vi "CalcParams.vi"(0 "Max":sgl, 5 "ClkRate":sgl, 7 "fc":sgl, 9 "deadtime":sgl) -> (4 "Parameters":T1={"max"=0.9999695, "Period"=0, "Deadtime"=1})   [LabVIEW 2015, in "SVPWMInterface.lvlib"]
doc: "Calculates parameters nescessary to configure the SPWM Core.\n\nClkRate - The clock rate in Hz that the core will execute at, typically determined by the clock rate of a single cycle timed loop. Typical values would be 40 MHz or 80 MHz. Recommended values would be 10 to 20 kHz.\n\nfc - Carrier frequency in Hz of the PWM. Recommended values would be 10 kHz to 20 kHz.\n\nDeadtime - Deadtime between switching between the Top and Bottom switch pairs in seconds."
uses:
  SVPWMInterface.lvlib
  SVPWM/SVPWM_SGL.ctl
  SVPWM/SVPWM.lvlib
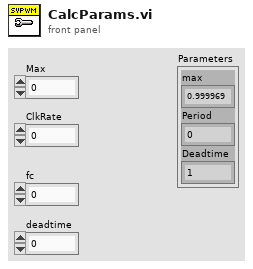
[diagram p1: front panel]
types:
  T1 = typedef "SVPWM.lvlib/SVPWM_SGL.ctl" = cluster{"max":sgl, "Period":u32, "Deadtime":u8}
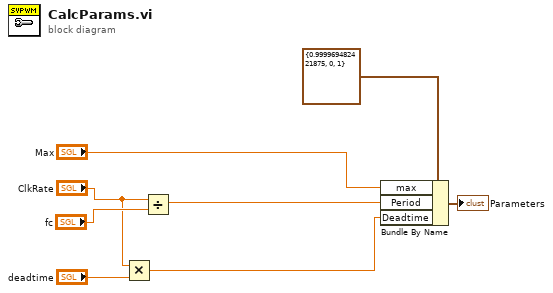
[diagram p0: block diagram]
diagram:
  n1 = Multiply(x="ClkRate", y="deadtime") -> (x*y=w2:sgl)
  n2 = Divide(x="ClkRate", y="fc") -> (x/y=w5:sgl)
  n3 = Bundle By Name(cluster=T1 {"max"=0.9999695, "Period"=0, "Deadtime"=1} ("SVPWM_SGL"), "max"="Max", "Period"=w5, "Deadtime"=w2) -> (→"Parameters":T1)
